vi "G#Debugger_CheckError.vi"(0 "refs":T1, 5 "error in (no error)":errorcluster) -> (19 "error out":errorcluster)   [LabVIEW 2017, in "G#Debugger.lvlib"]
uses:
  <vilib>/addons/_AddQ/G#Debugger/G#Debugger.lvlib
  <vilib>/addons/_AddQ/G#Debugger/private/G#Debugger_Refs.ctl
  <vilib>/addons/_AddQ/G#Object/utils/G#Object_ClassInfoType.ctl
  <vilib>/addons/_AddQ/G#Object/G#Object.lvclass
  <vilib>/addons/_AddQ/G#Object/utils/G#Object_ObjectInfoType.ctl
  <vilib>/addons/_AddQ/G#Object/utils/G#Object_CreateMethod.ctl
  <vilib>/addons/_AddQ/G#Debugger/private/G#Debugger_SubPanelInfo.ctl
  <vilib>/addons/_AddQ/G#Object/utils/G#Object_ClassHierarchy.ctl
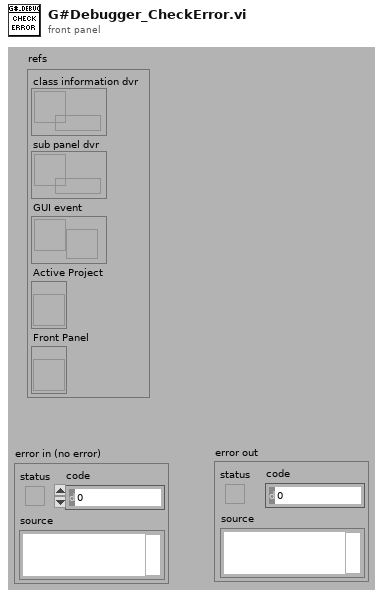
[diagram p1: front panel]
types:
  T1 = typedef "G#Debugger.lvlib/G#Debugger_Refs.ctl" = cluster{"class information dvr":refnum<data-value>, "sub panel dvr":refnum<data-value>, "GUI event":refnum<user-event>, "Active Project":refnum<vi>, "Front Panel":refnum<vi>}
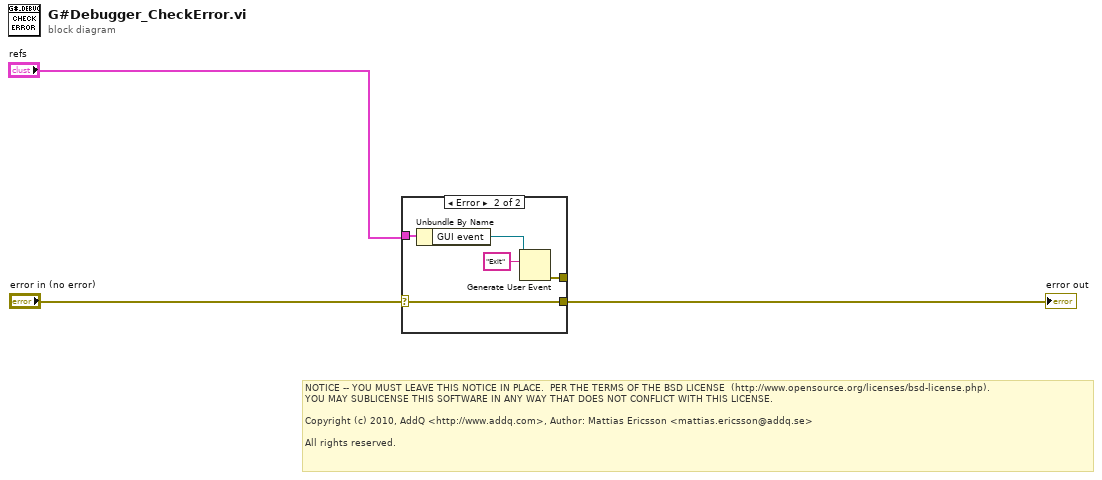
[diagram p0: block diagram]
diagram:
  # "NOTICE -- YOU MUST LEAVE THIS NOTICE IN PLACE.  PER THE TERMS OF THE BSD LICENSE  (http://www.opensource.org/licenses/bsd-license.php).\nYOU MAY SUBLICENSE THIS SOFTWARE IN ANY WAY THAT DOES NOT CONFLICT WITH THIS LICENSE.\n\nCopyright (c) 2010, AddQ <http://www.addq.com>, Author: Mattias Ericsson <mattias.ericsson@addq.se>\n\nAll rights reserved."
  n1 = case shown="Error" "error in (no error)" {
    selector: "error in (no error)" -> [w4 w9]
    tunnel: [w4 w9] -> w3
    tunnel: "refs" -> [_ w7]
    tunnel: [_ w5] -> _
    frame No Error {
    }
    frame Error {
      n2 = Unbundle By Name(w7) -> ("GUI event"=w6:refnum<user-event>)
      n3 = Generate User Event(user event=w6, event data cluster="Exit" ("event data")) -> (error out=w5:errorcluster)  [unwired: 2 in, 1 out]
    }
  }
  "error out" <- w3
